vi "Find Library in Project.vi"(9 "DQMH Modules Refs":refnum<vi>[](array[refnum]), 10 "Project Ref":refnum<vi>, 11 "DQMH Lib Ref":refnum<vi>) -> (0 "error out":errorcluster)   [LabVIEW 2019, in "Panther Dashboard.lvlib"]
uses:
  Panther Dashboard.lvlib
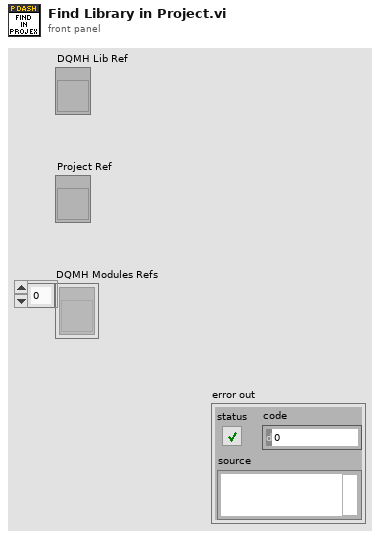
[diagram p1: front panel]
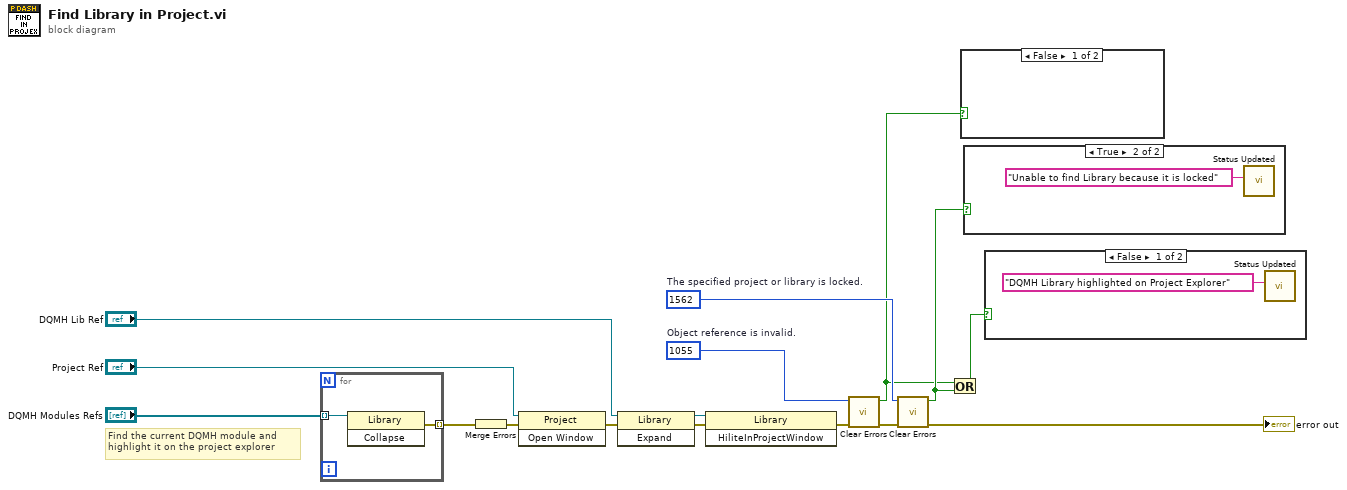
[diagram p0: block diagram]
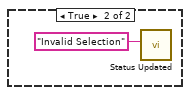
[diagram p4: hidden frame]
diagram:
  w4 = 1562  # The specified project or library is locked.
  w8 = 1055  # Object reference is invalid.
  # "Find the current DQMH module and\nhighlight it on the project explorer"
  n1 = for {
    tunnel: "DQMH Modules Refs" -> [w17] mode=indexing
    tunnel: [w18] -> w10 mode=indexing
    n2 = invoke class="Library" method="Collapse"(reference=w17) -> (error out=w18:errorcluster)  [unwired: 2 in, 2 out]
  }
  n3 = Merge Errors(w10) -> (w15:errorcluster)
  n4 = invoke class="Project" method="Open Window"(reference="Project Ref", error in=w15) -> (error out=w14:errorcluster)  [unwired: 1 in, 2 out]
  n5 = invoke class="Library" method="Expand"(reference="DQMH Lib Ref", error in=w14) -> (reference out=w9:refnum<vi>, error out=w13:errorcluster)  [unwired: 1 in, 1 out]
  n6 = invoke class="Library" method="HiliteInProjectWindow"(reference=w9, error in=w13) -> (error out=w16:errorcluster)  [unwired: 1 in, 2 out]
  n7 = call <vilib>:"Clear Errors.vi"("error in (no error)"=w16, "specific error code to clear (0: all)"=w8) -> ("error out"=w12:errorcluster, "specific error cleared?"=w2:bool)  [unwired: 4 in]
  n8 = call <vilib>:"Clear Errors.vi"("error in (no error)"=w12, "specific error code to clear (0: all)"=w4) -> ("error out"=→"error out":errorcluster, "specific error cleared?"=w3:bool)  [unwired: 4 in]
  n9 = Or(x=w2, y=w3) -> (x .or. y?=w1:bool)
  n10 = case shown="False" w2 {
    frame False {
    }
    frame True {
      n11 = call "Status Updated.vi"("Status"="Invalid Selection") -> ()  [unwired: 10 in, 1 out]
    }
  }
  n12 = case shown="True" w3 {
    frame False {
    }
    frame True {
      n13 = call "Status Updated.vi"("Status"="Unable to find Library because it is locked") -> ()  [unwired: 10 in, 1 out]
    }
  }
  n14 = case shown="False" w1 {
    frame False {
      n15 = call "Status Updated.vi"("Status"="DQMH Library highlighted on Project Explorer") -> ()  [unwired: 10 in, 1 out]
    }
    frame True {
    }
  }
